vi "CfgFile Write Configuration File.vi"(8 "error in (no error)":errorcluster, 10 "Configuration":T1={"Language"={"Name"=""}, "Path Config"={"Data Folder Path"=path "", "PNG Folder Path"=path "", "mp3 Folder Path"=path ""}, "Image Viewer Config"={"Center Point"={"Size"=3, "Color"=0, "Show?"=FALSE}, "bp Point"={"Size"=3, "Color"=0, "Show?"=FALSE}, "w Point"={"Size"=3, "Color"=0, "Show?"=FALSE}, "b Box"={"Fill Color"=0, "Border Color"=0, "Show?"=FALSE}, "i Box"={"Fill Color"=0, "Border Color"=0, "Show?"=FALSE}, "o Point"={"Size"=3, "Color"=0, "Show?"=FALSE}, "c Point"={"Size"=3, "Color"=0, "Show?"=FALSE}}}, 11 "LF2R IDE in":refnum<class "Main Panel.lvclass">) -> (0 "error out":errorcluster, 3 "LF2R IDE out":refnum<class "Main Panel.lvclass">)   [LabVIEW 2018, in "Main Panel.lvlib" / "Main Panel.lvclass"]
uses:
  Main Panel.lvclass
  Const Configuration.ctl
  Const Path Setting.ctl
  Const Image Viewer Setting.ctl
  13bfee12-6dc2-484c-8d8d-985dc1fbf3c4.vi
  <vilib>/JDP Science/JSONtext/Variant to JSON Text.vi
  <vilib>/JDP Science/JSONtext/LVClass Serializer/JSONtext LVClass Serializer.lvclass
  <vilib>/JDP Science/JSONtext/JSONtext.lvlib
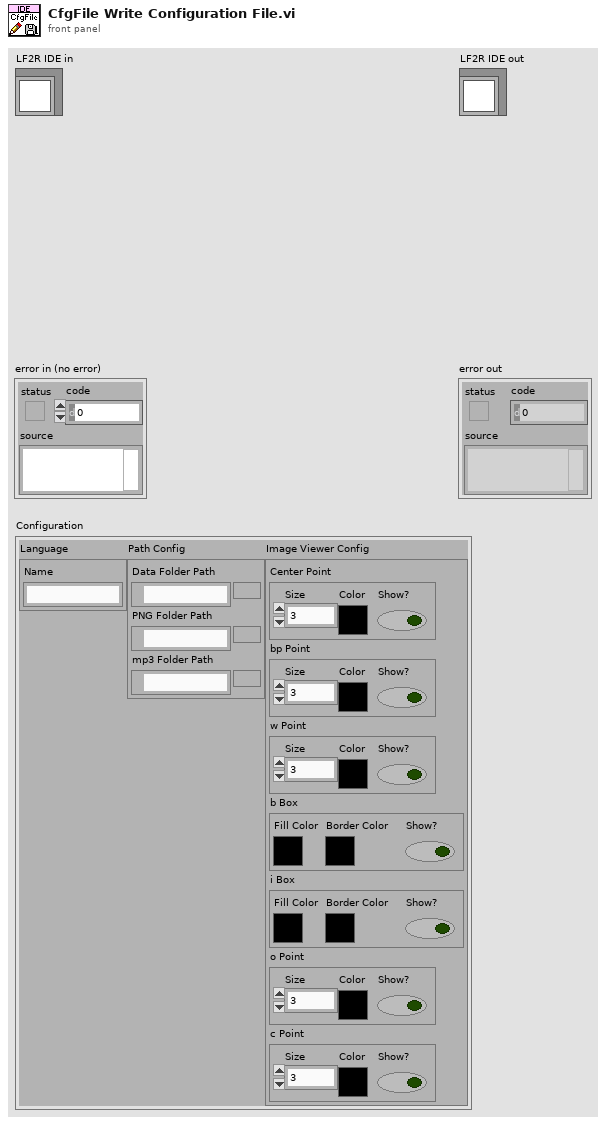
[diagram p1: front panel]
types:
  T1 = typedef "Main Panel.lvlib/Main Panel.lvclass/Const Configuration.ctl" = cluster{"Language":cluster{"Name":string}, "Path Config":T2, "Image Viewer Config":T3}
  T2 = typedef "Main Panel.lvlib/Main Panel.lvclass/Const Path Setting.ctl" = cluster{"Data Folder Path":path, "PNG Folder Path":path, "mp3 Folder Path":path}
  T3 = typedef "Main Panel.lvlib/Main Panel.lvclass/Const Image Viewer Setting.ctl" = cluster{"Center Point":cluster{"Size":i32, "Color":u32, "Show?":bool}, "bp Point":cluster{"Size":i32, "Color":u32, "Show?":bool}, "w Point":cluster{"Size":i32, "Color":u32, "Show?":bool}, "b Box":cluster{"Fill Color":u32, "Border Color":u32, "Show?":bool}, "i Box":cluster{"Fill Color":u32, "Border Color":u32, "Show?":bool}, "o Point":cluster{"Size":i32, "Color":u32, "Show?":bool}, "c Point":cluster{"Size":i32, "Color":u32, "Show?":bool}}
  T4 = enum16{"open", "replace", "create", "open or create", "replace or create", "replace or create with confirmation"}
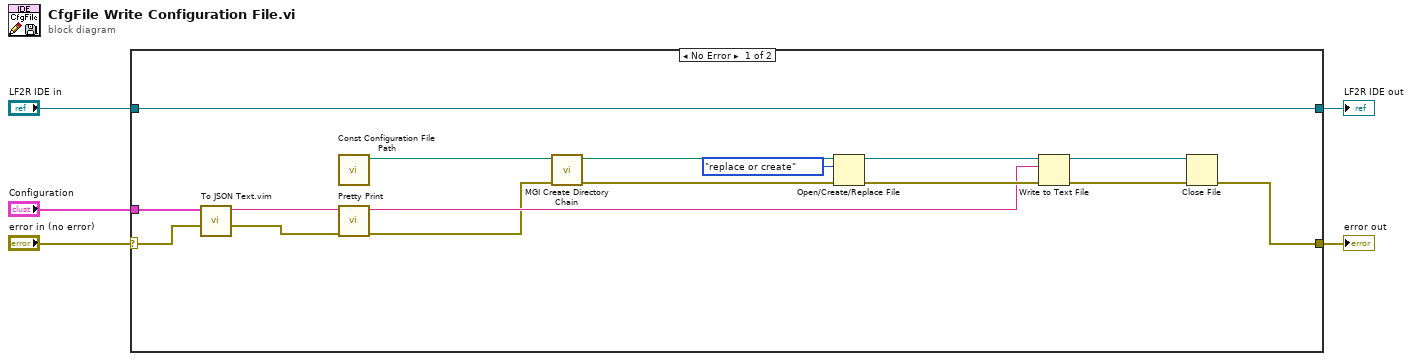
[diagram p0: block diagram]
diagram:
  n1 = case shown="No Error" "error in (no error)" {
    selector: "error in (no error)" -> [w11 w23]
    tunnel: [w10 w23] -> w4
    tunnel: [w13 w22] -> w2
    tunnel: "LF2R IDE in" -> [w13 w22]
    tunnel: "Configuration" -> [w12 _]
    frame No Error {
      n2 = call "To JSON Text.vim"("error in (no error)"=w11, "Anything"=w12) -> ("error out"=w6:errorcluster, "<JSON>"=w9:string)  [unwired: 8 in]
      n3 = call "Const Configuration File Path.vi"() -> ("Config File Path"=w15:path)  [unwired: 11 in]
      n4 = call <vilib>:"Pretty Print.vi"("error in (no error)"=w6, "JSON"=w9) -> ("error out"=w7:errorcluster, "<JSON>"=w8:string)  [unwired: 7 in, 1 out]
      n5 = call <userlib>:"MGI Create Directory Chain.vi"("Error In"=w7, "Path"=w15) -> ("Error Out"=w20:errorcluster, "Duplicate Path"=w21:path)  [unwired: 8 in]
      n6 = Open/Create/Replace File(file path (use dialog)=w21, error in=w20, operation (0:open)=T4."replace or create") -> (refnum out=w19:refnum<file>, error out=w18:errorcluster)  [unwired: 3 in, 1 out]
      n7 = Write to Text File(file (use dialog)=w19, text=w8, error in=w18) -> (refnum out=w17:refnum<file>, error out=w16:errorcluster)  [unwired: 1 in, 1 out]
      n8 = Close File(refnum=w17, error in=w16) -> (error out=w10:errorcluster)  [unwired: 1 out]
    }
    frame Error {
    }
  }
  "error out" <- w4
  "LF2R IDE out" <- w2
